vi "MotionProfiling_2D_PushPointViaCTRE.vi"(7 "Motion Profile Status":T6, 8 "CusorIn":u32, 9 "NumberOfPointsInArray":i32, 10 "ArrayIn":dbl[][](array[numeric]), 11 "PhoenixMotorControlDevRef":T1={"DeviceStatus"={"status"=FALSE, "code"=0, "source"=""}, "Type"=enum."PWM", "PWM"={"PWM Channel"=enum."Invalid", "DeadBand"={"Name"="", "maxPositivePwm"=0, "minPositivePwm"=0, "centerPwm"=0, "maxNegativePwm"=0, "minNegativePwm"=0, "angularRange"=0}}, "CAN"={"Device Number"=0, "SetOutput VI Ref"=variant(enum8{"Percent VBus", "Current", "Speed", "Position", "Voltage"} enum."Percent VBus"), "GetOutput VI Ref"=variant(refnum<k1> refnum), "Enable VI Ref"=variant(dbl 12.0), "Disable VI Ref"=variant(enum8{"Percent VBus", "Speed", "Position", "Slave", "Unchanged / Invalid", "Voltage Compensation", "Current", "Motion Profile"} enum."Percent VBus"), "Data"=variant}, "Invert"=FALSE, "DIO PWM"={"PWM \"Enable\" Channel"=enum."Invalid", "DIOChannel"=enum."Invalid", "PWM Rate"=0.0}}) -> (0 "CursorOut":u32, 3 "PhoenixMotorControlDevRef 2":T1={"DeviceStatus"={"status"=FALSE, "code"=0, "source"=""}, "Type"=enum."PWM", "PWM"={"PWM Channel"=enum."Invalid", "DeadBand"={"Name"="", "maxPositivePwm"=0, "minPositivePwm"=0, "centerPwm"=0, "maxNegativePwm"=0, "minNegativePwm"=0, "angularRange"=0}}, "CAN"={"Device Number"=0, "SetOutput VI Ref"=variant, "GetOutput VI Ref"=variant, "Enable VI Ref"=variant, "Disable VI Ref"=variant, "Data"=variant}, "Invert"=FALSE, "DIO PWM"={"PWM \"Enable\" Channel"=enum."Invalid", "DIOChannel"=enum."Invalid", "PWM Rate"=0.0}})   [LabVIEW 2017]
uses:
  <vilib>/Rock Robotics/WPI/MotorControl/WPI_MotorControlDeviceRef.ctl
  <vilib>/Rock Robotics/WPI/MotorControl/WPI_MotorControlType.ctl
  <vilib>/Rock Robotics/SystemInterfaces/DIO/FPGA_DIOPWMChannel.ctl
  <vilib>/Rock Robotics/WPI/PWM/WPI_PWMDeadband.ctl
  <vilib>/Rock Robotics/SystemInterfaces/DIO/FPGA_DIOChannel.ctl
  <vilib>/Rock Robotics/WPI/ThirdParty/Phoenix-LabVIEW/Motor Controller/Controls/CTRE_Phoenix_MotorControl_TrajectoryPointTimeDur.ctl
  Constants.vi
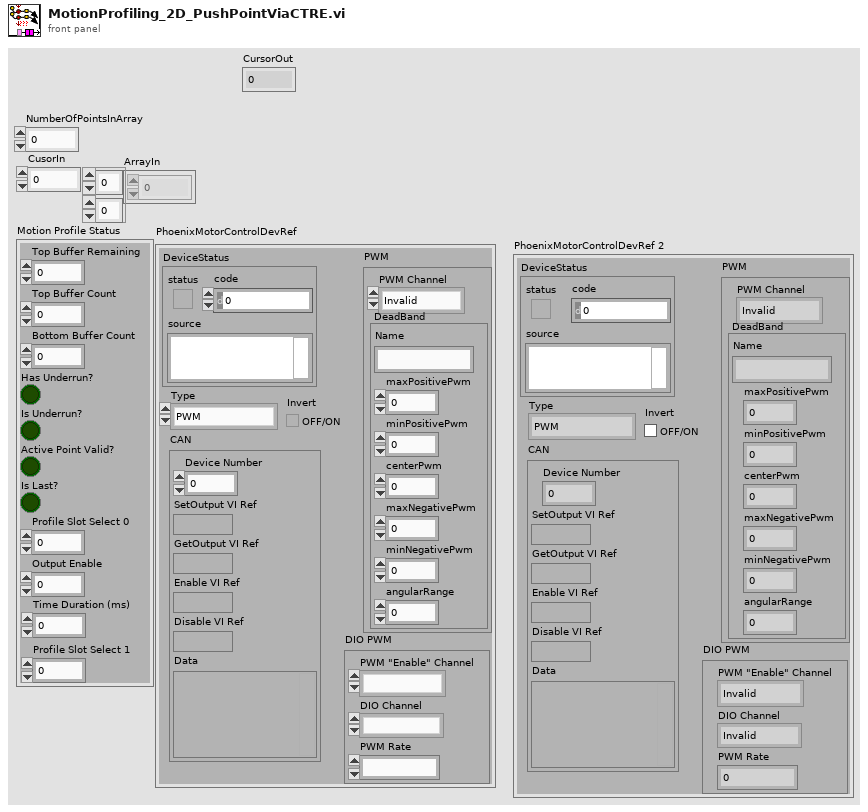
[diagram p1: front panel]
types:
  T1 = typedef "WPI_MotorControlDeviceRef.ctl" = cluster{"DeviceStatus":errorcluster, "Type":T2, "PWM":cluster{"PWM Channel":T3, "DeadBand":T4}, "CAN":cluster{"Device Number":u8, "SetOutput VI Ref":variant, "GetOutput VI Ref":variant, "Enable VI Ref":variant, "Disable VI Ref":variant, "Data":variant}, "Invert":bool, "DIO PWM":cluster{"PWM \"Enable\" Channel":T3, "DIOChannel":T5, "PWM Rate":dbl}}
  T2 = typedef "WPI_MotorControlType.ctl" = enum16{"PWM", "CAN", "DIO PWM"}
  T3 = typedef "FPGA_DIOPWMChannel.ctl" = enum8{"PWM 0", "PWM 1", "PWM 2", "PWM 3", "PWM 4", "PWM 5", "PWM 6", "PWM 7", "PWM 8", "PWM 9", "PWM MXP 0", "PWM MXP 1", "PWM MXP 2", "PWM MXP 3", "PWM MXP 4", "PWM MXP 5", "PWM MXP 6", "PWM MXP 7", "PWM MXP 8", "PWM MXP 9", "Invalid"}
  T4 = typedef "WPI_PWMDeadband.ctl" = cluster{"Name":string, "maxPositivePwm":i32, "minPositivePwm":i32, "centerPwm":i32, "maxNegativePwm":i32, "minNegativePwm":i32, "angularRange":u16}
  T5 = typedef "FPGA_DIOChannel.ctl" = enum8{"DIO 0", "DIO 1", "DIO 2", "DIO 3", "DIO 4", "DIO 5", "DIO 6", "DIO 7", "DIO 8", "DIO 9", "DIO MXP 0", "DIO MXP 1", "DIO MXP 2", "DIO MXP 3", "DIO MXP 4", "DIO MXP 5", "DIO MXP 6", "DIO MXP 7", "DIO MXP 8", "DIO MXP 9", "DIO MXP 10", "DIO MXP 11", "DIO MXP 12", "DIO MXP 13", "DIO MXP 14", "DIO MXP 15", "SPI Port CS1", "SPI Port CS2", "SPI Port CS3", "SPI Port MISO", "SPI Port MOSI", "Invalid"}
  T6 = cluster{"Top Buffer Remaining":i32, "Top Buffer Count":i32, "Bottom Buffer Count":i32, "Has Underrun?":bool, "Is Underrun?":bool, "Active Point Valid?":bool, "Is Last?":bool, "Profile Slot Select 0":i32, "Output Enable":i32, "Time Duration (ms)":i32, "Profile Slot Select 1":i32}
  T7 = typedef "CTRE_Phoenix_MotorControl_TrajectoryPointTimeDur.ctl" = i32
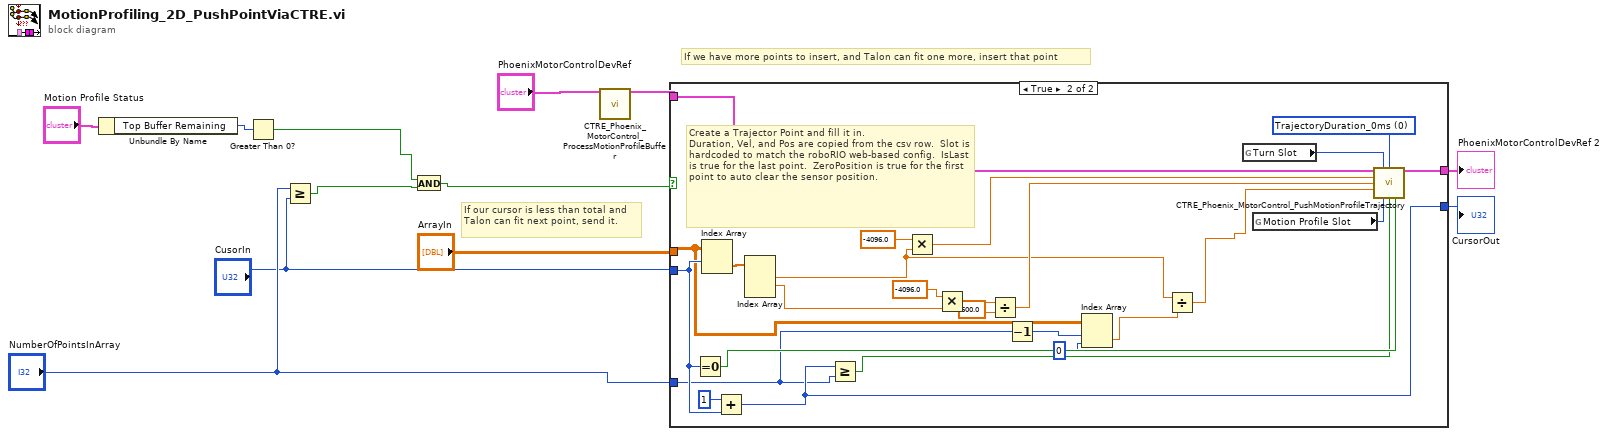
[diagram p0: block diagram]
diagram:
  # "If our cursor is less than total and Talon can fit next point, send it."
  # "If we have more points to insert, and Talon can fit one more, insert that point"
  n1 = Unbundle By Name("Motion Profile Status") -> ("Top Buffer Remaining"=w9:i32)
  n2 = Greater Than 0?(x=w9) -> (x > 0?=w7:bool)
  n3 = Greater Or Equal?(x="NumberOfPointsInArray", y="CusorIn") -> (x >= y?=w6:bool)
  n4 = And(x=w7, y=w6) -> (x .and. y?=w5:bool)
  n5 = call <vilib>:"CTRE_Phoenix_MotorControl_ProcessMotionProfileBuffer.vi"("PhoenixMotorControlDevRef"="PhoenixMotorControlDevRef") -> ("PhoenixMotorControlDevRef"=w12:T1)  [unwired: 13 in, 1 out]
  n6 = case shown="True" w5 {
    tunnel: "ArrayIn" -> [_ w25]
    tunnel: [w14 w36] -> w1
    tunnel: "CusorIn" -> [w14 w37]
    tunnel: "NumberOfPointsInArray" -> [_ w21]
    tunnel: w12 -> [w13 w35]
    tunnel: [w13 w16] -> w3
    frame False {
    }
    frame True {
      w27 = T7 0 items=["TrajectoryDuration_0ms"=0, "TrajectoryDuration_5ms"=5, "TrajectoryDuration_10ms"=10, "TrajectoryDuration_20ms"=20, "TrajectoryDuration_30ms"=30, "TrajectoryDuration_40ms"=40, "TrajectoryDuration_50ms"=50, "TrajectoryDuration_100ms"=100] ("durationMs")
      # "Create a Trajector Point and fill it in.\nDuration, Vel, and Pos are copied from the csv row.  Slot is hardcoded to match the roboRIO web-based config.  IsLast is true for the last point.  ZeroPosition is true for the first point to auto clear the sensor position."
      n7 = Equal To 0?(x=w37) -> (x = 0?=w34:bool)
      n8 = Index Array(array=w25, index (row)=w37) -> (element=w38:dbl[])  [unwired: 1 in]
      n9 = Add(x=u32 1, y=w37) -> (x+y=w36:u32)
      n10 = Index Array(array=w38) -> (element #1=w19:dbl, element #2=w31:dbl)  [unwired: 3 in, 1 out]
      n11 = Greater Or Equal?(x=w36, y=w21) -> (x >= y?=w33:bool)
      n12 = Multiply(x=-4096.0, y=w19) -> (x*y=w22:dbl)
      n13 = Multiply(x=-4096.0, y=w31) -> (x*y=w29:dbl)
      n14 = Divide(x=w29, y=600.0) -> (x/y=w28:dbl)
      n15 = Decrement(x=w21) -> (x-1=w20:i32)
      n16 = Index Array(array=w25, index (row)=w20, index (col)=0 ("disabled index (col)")) -> (element=w23:dbl)
      n17 = Divide(x=w19, y=w23) -> (x/y=w15:dbl)
      n18 = global read "Constants.vi" "Turn Slot"() -> (w17:i32)
      n19 = global read "Constants.vi" "Motion Profile Slot"() -> (w18:i32)
      n20 = call <vilib>:"CTRE_Phoenix_MotorControl_PushMotionProfileTrajectory.vi"("PhoenixMotorControlDevRef"=w35, "profileSlotSelect1"=w17, "durationMs"=w27, "position"=w22, "velocity"=w28, "auxiliaryPos"=w15, "profileSlotSelect0"=w18, "isLastPoint?"=w33, "Zero Position?"=w34) -> ("PhoenixMotorControlDevRef"=w16:T1)  [unwired: 5 in, 1 out]
    }
  }
  "PhoenixMotorControlDevRef 2" <- w3
  "CursorOut" <- w1
